vi "3일차3vi.vi"() -> ()   [LabVIEW 2014]
uses:
  <vilib>/Analysis/NI_AALBase.lvlib
panel:
  out "웨이브폼 그래프":dbl[](graph)
  in  "정지":bool
  in  "삼각":bool
  in  "SINE":bool
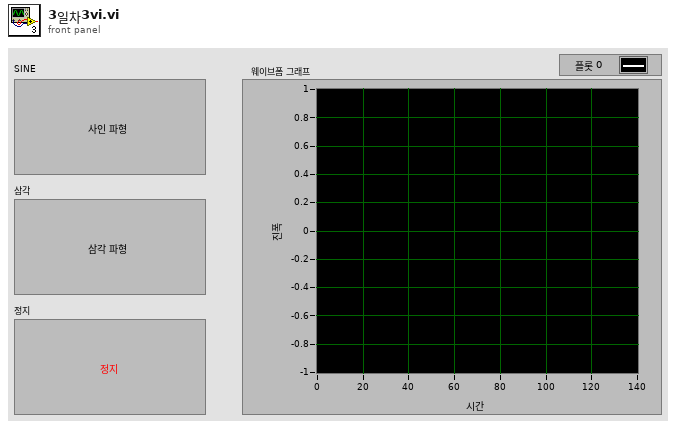
[diagram p1: front panel]
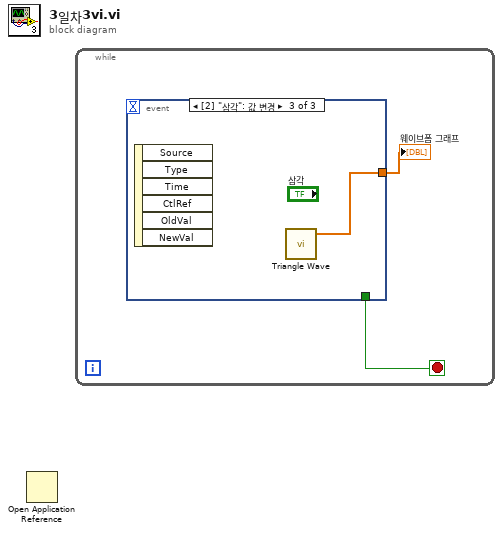
[diagram p0: block diagram]
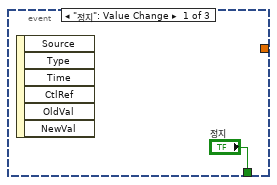
[diagram p2: hidden frame]
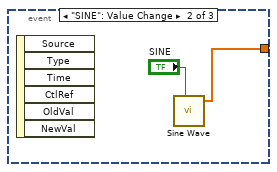
[diagram p3: hidden frame]
diagram:
  n1 = Open Application Reference() -> ()  [unwired: 4 in, 2 out]
  n2 = while {
    stop <- w2 stop-if-true
    n3 = event shown="[2] \"삼각\": 값 변경" {
      selector: _ -> [_ _ _]
      dyn-events: _ -> [_ _ _]
      timeout: _ -> [_ _ _]
      tunnel: ["정지" _ _] -> w2
      tunnel: [_ w4 w6] -> w1
      event "정지": Value Change {
        n4 = event-data() -> ()  [unwired: 1 in, 6 out]
      }
      event "SINE": Value Change {
        n5 = event-data() -> ()  [unwired: 1 in, 6 out]
        n6 = call <vilib>:"Sine Wave.vi"("reset phase"="SINE") -> ("sine wave"=w4:dbl[])  [unwired: 4 in, 2 out]
      }
      event "삼각": Value Change {
        n7 = event-data() -> ()  [unwired: 1 in, 6 out]
        n8 = call <vilib>:"Triangle Wave.vi"() -> ("triangle wave"=w6:dbl[])  [unwired: 5 in, 2 out]
      }
    }
    "웨이브폼 그래프" <- w1
  }
